vi "InitStateQueue.vi"(7 "QueueMaxNumber":i32=-1, 8 "error in (no error)":errorcluster, 9 "States":T2=enum."TestSequence", 11 "Slot":T1) -> (0 "error out":errorcluster, 3 "QueueOut":variant)   [LabVIEW 2013]
uses:
  SysControl/States.ctl
  SysControl/Slot.ctl
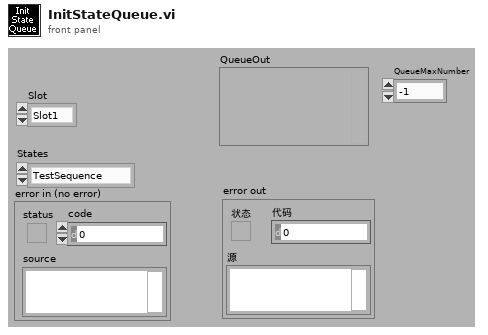
[diagram p1: front panel]
types:
  T1 = typedef "Slot.ctl" = enum16{"Slot1", "Slot2", "Slot3", "Slot4"}
  T2 = typedef "States.ctl" = enum16{"Init", "PreUUT", "Idle", "SetUp", "TestSequence", "PostUUT", "StopTest", "Debug Mode", "Selection Mode", "Loop Mode", "Error", "Wait"}
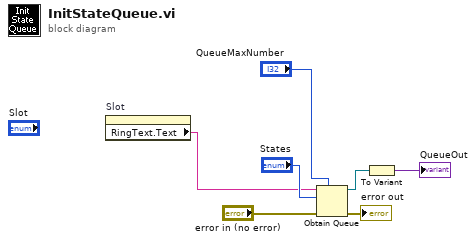
[diagram p0: block diagram]
diagram:
  n1 = property on="Slot" class="Enum (严格)"() -> ("RingText.Text"=w1:string)  [unwired: 2 in, 2 out]
  n2 = Obtain Queue(max queue size (-1, unlimited)="QueueMaxNumber", name (unnamed)=w1, element data type="States", error in (no error)="error in (no error)") -> (queue out=w6:refnum<queue>, error out=→"error out":errorcluster)  [unwired: 1 in, 1 out]
  n3 = To Variant(anything=w6) -> (Variant=→"QueueOut":variant)
